vi "Write Trigger.vi"(8 "error in (no error)":errorcluster, 10 "Trigger":u16(ring) items=["Internal", "External", "-", "-", "-", "-", "External Start"], 11 "CCDCamera in":refnum<class "Simulated_CCD_Camera.lvclass">) -> (0 "error out":errorcluster, 3 "CCDCamera out":refnum<class "Simulated_CCD_Camera.lvclass">)   [LabVIEW 2018, in "Simulated_CCD_Camera.lvclass"]
uses:
  Simulated_CCD_Camera.lvclass
  Simulated_CCD_Camera.lvclass/Simulated_CCD_Camera.ctl
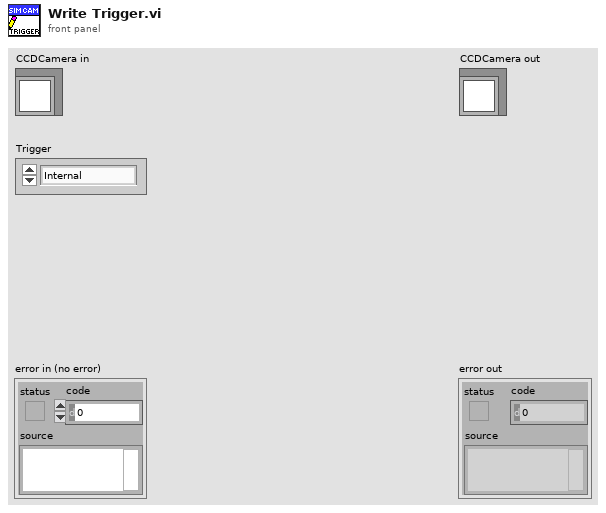
[diagram p1: front panel]
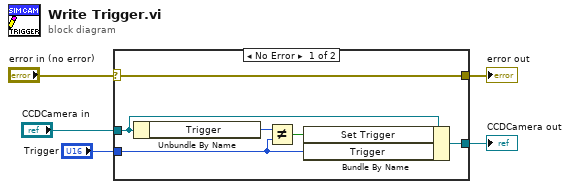
[diagram p0: block diagram]
diagram:
  n1 = case shown="No Error" "error in (no error)" {
    selector: "error in (no error)" -> [w11 w12]
    tunnel: [w11 w12] -> w4
    tunnel: [w10 w13] -> w2
    tunnel: "CCDCamera in" -> [w9 w13]
    tunnel: "Trigger" -> [w7 _]
    frame No Error {
      n2 = Unbundle By Name(w9) -> ("Trigger"=w8:u16)
      n3 = Not Equal?(x=w8, y=w7) -> (x != y?=w6:bool)
      n4 = Bundle By Name(cluster=w9, "Set Trigger"=w6, "Trigger"=w7) -> (w10:refnum<class "Simulated_CCD_Camera.lvclass">)
    }
    frame Error {
    }
  }
  "error out" <- w4
  "CCDCamera out" <- w2
